vi "xy data array moving average (subVI).vi"(10 "window size (3)":u32=3, 11 "xy chart data []":cluster{"x":dbl[], "y":dbl[]}[](array[cluster])) -> (3 "xy chart data smooth []":cluster{"x":dbl[], "y":dbl[]}[](array[cluster]))   [LabVIEW 2021]
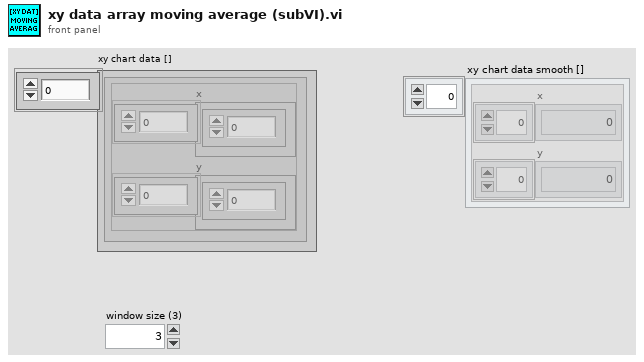
[diagram p1: front panel]
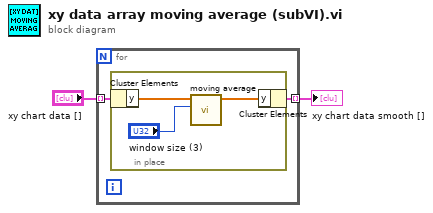
[diagram p0: block diagram]
diagram:
  n1 = for {
    tunnel: "xy chart data []" -> [w4] mode=indexing
    tunnel: [w3] -> w1 mode=indexing
    n2 = in-place {
      n3 = in-place-cluster #1(w4) -> ("y"=w7:dbl[])
      n4 = call "moving average.vi"("window size (3)"="window size (3)", "x"=w7) -> ("x smoothed"=w6:dbl[])  [unwired: 8 in, 1 out]
      n5 = in-place-cluster #1("y"=w6) -> (w3:cluster{"x":dbl[], "y":dbl[]})
    }
  }
  "xy chart data smooth []" <- w1
